vi "ExpValidateExperimentFile.vi"(9 "AsSubCaller":bool, 11 "Experiment file path (or root calling vi)":path) -> (2 "Found?":bool, 3 "Experiment File path":path)   [LabVIEW 2017]
uses:
  <userlib>/_OpenG.lib/file/file.llb/Strip Path Extension - Path__ogtk.vi
  <userlib>/_OpenG.lib/file/file.llb/File Exists - Scalar__ogtk.vi
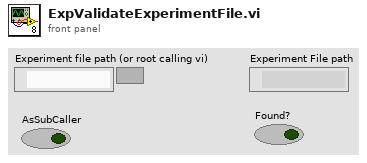
[diagram p1: front panel]
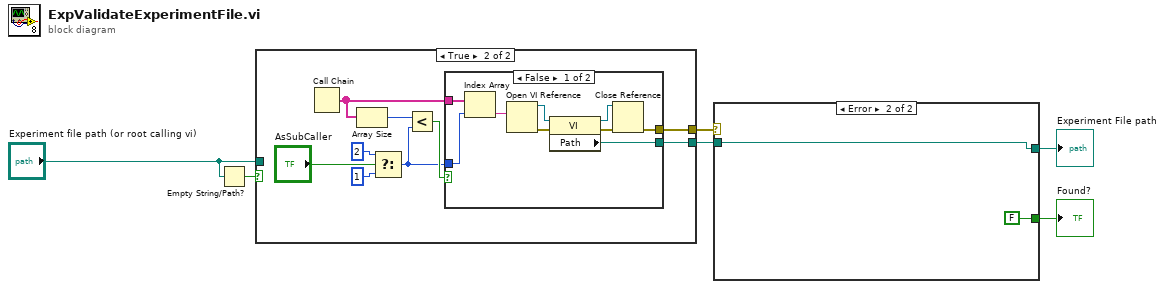
[diagram p0: block diagram]
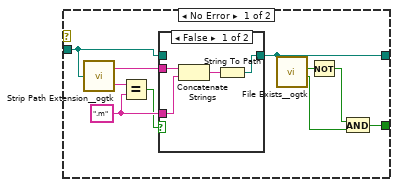
[diagram p2: hidden frame]
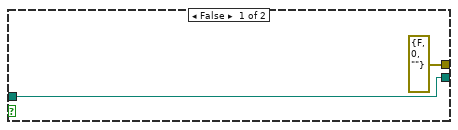
[diagram p4: hidden frame]
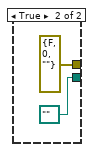
[diagram p5: hidden frame]
diagram:
  n1 = Empty String/Path?(string/path="Experiment file path (or root calling vi)") -> (empty?=w3:bool)
  n2 = case shown="True" w3 {
    tunnel: "Experiment file path (or root calling vi)" -> [w8 _]
    tunnel: [w8 w14] -> w4
    tunnel: [errorcluster {"status"=FALSE, "code"=0, "source"=""} ("error out") w13] -> w6
    frame False {
    }
    frame True {
      n3 = Call Chain() -> (call chain=w17:string[])
      n4 = Array Size(array=w17) -> (size(s)=w16:i32)
      n5 = Select(t=2 ("y"), s="AsSubCaller", f=1 ("y")) -> (s? t:f=w9:i32)
      n6 = Less?(x=w16, y=w9) -> (x < y?=w15:bool)
      n7 = case shown="False" w15 {
        tunnel: w17 -> [w26 _]
        tunnel: [w25 path ""] -> w14
        tunnel: [w20 errorcluster {"status"=FALSE, "code"=0, "source"=""} ("error out")] -> w13
        tunnel: w9 -> [w19 _]
        frame False {
          n8 = Index Array(array=w26, index=w19) -> (element=w18:string)
          n9 = Open VI Reference(vi path=w18) -> (vi reference=w24:refnum<vi>, error out=w22:errorcluster)  [unwired: 5 in]
          n10 = property class="VI"(reference=w24, error in=w22) -> (reference out=w23:refnum<vi>, error out=w21:errorcluster, "Path"=w25:path)
          n11 = Close Reference(reference=w23, error in (no error)=w21) -> (error out=w20:errorcluster)
        }
        frame True {
        }
      }
    }
  }
  n12 = case shown="Error" w6 {
    tunnel: [w35 FALSE] -> w1
    tunnel: w4 -> [w30 w45]
    tunnel: [w29 w45] -> w5
    frame No Error {
      w33 = ".m" ("string")
      n13 = call-poly <userlib>:"Strip Path Extension__ogtk.vi"("path"=w30) -> ("root"=w34:string, "extension"=w32:string)
      n14 = Equal?(x=w32, y=w33) -> (x = y?=w31:bool)
      n15 = case shown="False" w31 {
        tunnel: [w42 w43] -> w29
        tunnel: w34 -> [w40 _]
        tunnel: w33 -> [w39 _]
        tunnel: w30 -> [_ w43]
        frame False {
          n16 = Concatenate Strings(w40, w39) -> (w41:string)
          n17 = String To Path(string=w41) -> (path=w42:path)
        }
        frame True {
        }
      }
      n18 = call-poly <userlib>:"File Exists__ogtk.vi"("file path"=w29) -> ("is directory"=w38:bool, "exists"=w37:bool)  [unwired: 6 in]
      n19 = Not(x=w38) -> (.not. x?=w36:bool)
      n20 = And(x=w36, y=w37) -> (x .and. y?=w35:bool)
    }
    frame Error {
    }
  }
  "Experiment File path" <- w5
  "Found?" <- w1
